vi "GetDiagramOutputs.vi"(6 "error in":errorcluster, 9 "ForLoop in":refnum<class "ForLoop.lvclass">) -> (0 "error out":errorcluster, 3 "ForLoop out":refnum<class "ForLoop.lvclass">, 4 "output terminals":refnum<class "Terminal.lvclass">[][](array[class]))   [LabVIEW 2014, in "ForLoop.lvclass"]
uses:
  ForLoop.lvclass
  Terminal/Terminal.lvclass
  ForLoop.lvclass/ForLoop.ctl
  Loop/Loop.lvclass/Loop.ctl
  Loop/Loop.lvclass
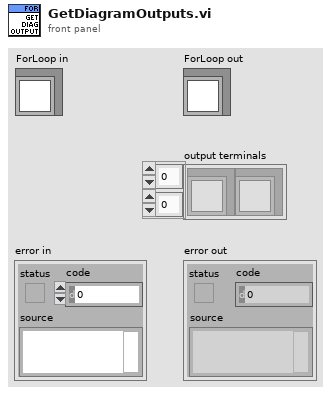
[diagram p1: front panel]
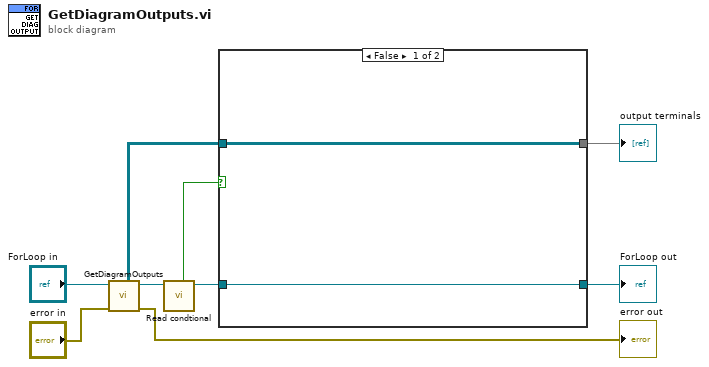
[diagram p0: block diagram]
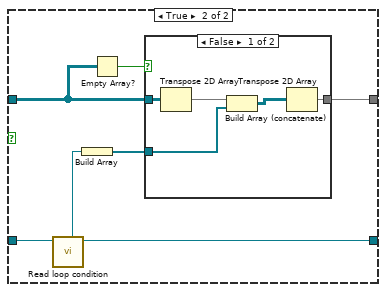
[diagram p2: hidden frame]
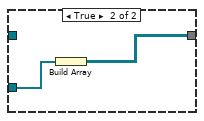
[diagram p3: hidden frame]
diagram:
  n1 = call-parent "GetDiagramOutputs.vi"("error in"="error in", "Loop in"="ForLoop in") -> ("error out"=→"error out":errorcluster, "Loop out"=w3:refnum<class "ForLoop.lvclass">, "output terminals"=w4:refnum<class "Terminal.lvclass">[][])  [unwired: 5 in]
  n2 = call "Read condtional.vi"("ForLoop in"=w3) -> ("ForLoop out"=w2:refnum<class "ForLoop.lvclass">, "condtional"=w1:bool)  [unwired: 7 in]
  n3 = case shown="False" w1 {
    tunnel: [w10 w18] -> w6
    tunnel: [w11 w16] -> w5
    tunnel: w4 -> [w11 w15]
    tunnel: w2 -> [w10 w13]
    frame False {
    }
    frame True {
      n4 = call "Read loop condition.vi"("Loop in"=w13) -> ("Loop out"=w18:refnum<class "ForLoop.lvclass">, "conditional terminal"=w12:refnum<class "Terminal.lvclass">)  [unwired: 7 in]
      n5 = Build Array(w12) -> (w17:refnum<class "Terminal.lvclass">[])
      n6 = Empty Array?(array=w15) -> (empty?=w14:bool)
      n7 = case shown="False" w14 {
        tunnel: [w19 w24] -> w16
        tunnel: w17 -> [w22 w25]
        tunnel: w15 -> [w21 _]
        frame False {
          n8 = Transpose 2D Array(2D array=w21) -> (transposed array=w20:refnum<class "Terminal.lvclass">[][])
          n9 = Build Array (concatenate)(w20, w22) -> (w23:refnum<class "Terminal.lvclass">[][])
          n10 = Transpose 2D Array(2D array=w23) -> (transposed array=w19:refnum<class "Terminal.lvclass">[][])
        }
        frame True {
          n11 = Build Array(w25) -> (w24:refnum<class "Terminal.lvclass">[][])
        }
      }
    }
  }
  "ForLoop out" <- w6
  "output terminals" <- w5
